vi "Configure Parameter.vi"(4 "value":u8[](array[numeric]), 6 "value byte count":u8(ring) items=["variable"=0, "1"=1, "2"=2, "4"=4], 7 "process number":u8=1, 8 "error in (no error)":errorcluster, 9 "parameter number":u8, 10 "node":u8, 11 "ProPar in":refnum<class "PL Bronkhorst ProPar.lvclass">) -> (0 "error out":errorcluster, 3 "ProPar out":refnum<class "PL Bronkhorst ProPar.lvclass">)   [LabVIEW 2015, in "PL Bronkhorst ProPar.lvclass"]
doc: "Configures specified <b>parameter</b> of the specified <b>node</b>."
uses:
  PL Bronkhorst ProPar.lvclass
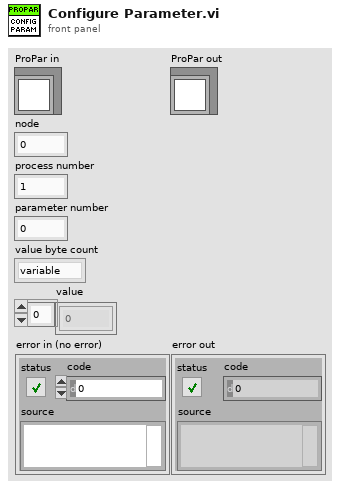
[diagram p1: front panel]
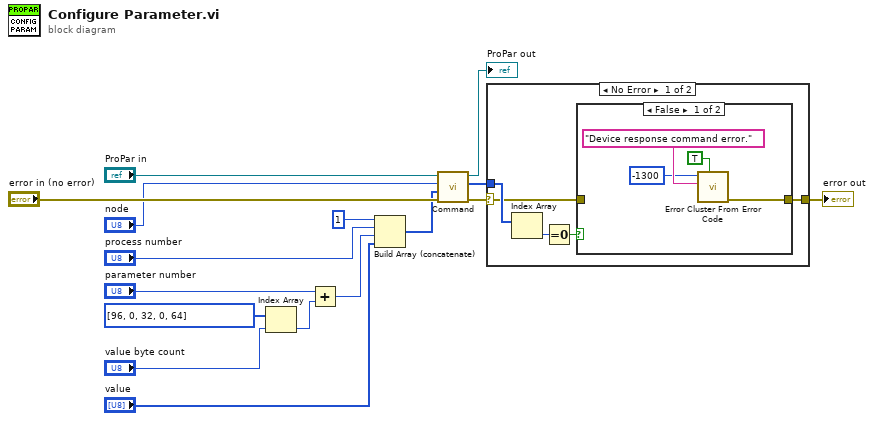
[diagram p0: block diagram]
diagram:
  n1 = Index Array(array=u8[] [96, 0, 32, 0, 64], index="value byte count") -> (element=w1:u8)
  n2 = Add(x="parameter number", y=w1) -> (x+y=w9:u8)
  n3 = Build Array (concatenate)(u8 1 ("node"), "process number", w9, "value") -> (w7:u8[])
  n4 = call "Command.vi"("error in (no error)"="error in (no error)", "command data"=w7, "node"="node", "ProPar in"="ProPar in") -> ("error out"=w6:errorcluster, "response data"=w4:u8[], "ProPar out"=→"ProPar out":refnum<class "PL Bronkhorst ProPar.lvclass">)  [unwired: 5 in]
  n5 = case shown="No Error" w6 {
    selector: w6 -> [w17 w27]
    tunnel: [w18 w27] -> w5
    tunnel: w4 -> [w19 _]
    frame No Error {
      n6 = Index Array(array=w19) -> (element=w21:u8)  [unwired: 1 in]
      n7 = Equal To 0?(x=w21) -> (x = 0?=w20:bool)
      n8 = case shown="False" w20 {
        tunnel: [w22 w26] -> w18
        tunnel: w17 -> [_ w26]
        frame False {
          n9 = call <vilib>:"Error Cluster From Error Code.vi"("show call chain? (False)"=TRUE, "error message (\"\")"="Device response command error." ("format string"), "error code (0)"=-1300) -> ("error out"=w22:errorcluster)  [unwired: 6 in]
        }
        frame True {
        }
      }
    }
    frame Error {
    }
  }
  "error out" <- w5
